vi "Read back eight strings from file.vi"(0 "File Path":path, 11 "error in (no error)":errorcluster) -> (2 "item 1":string, 3 "item 2":string, 4 "item 3":string, 6 "item 4":string, 8 "item 5":string, 10 "item 6":string, 13 "item 8":string, 14 "item 7":string, 15 "error out":errorcluster)   [LabVIEW 2013]
uses:
  <vilib>/Utility/file.llb/Read From Spreadsheet File (string).vi
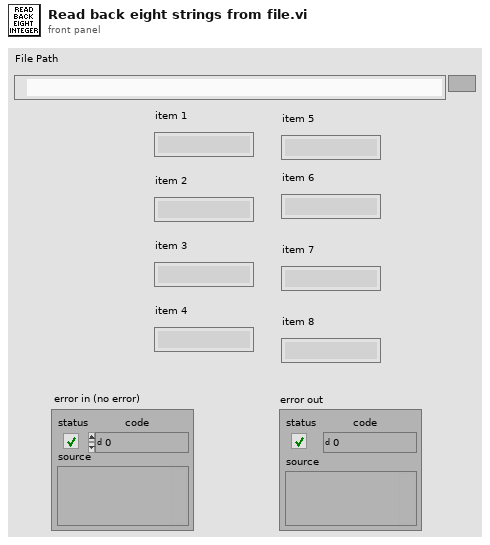
[diagram p1: front panel]
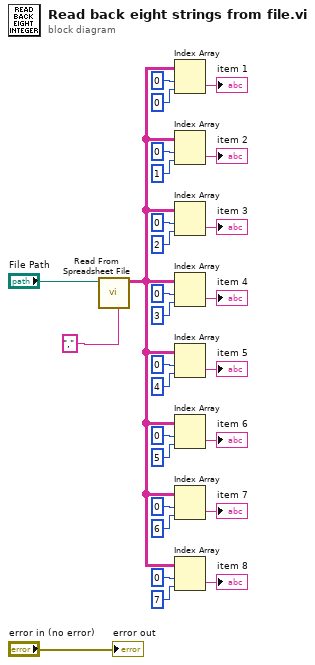
[diagram p0: block diagram]
diagram:
  n1 = call-poly <vilib>:"Read From Spreadsheet File.vi"("delimiter (\\t)"="," ("delimiter (\\t)"), "file path (dialog if empty)"="File Path") -> ("all rows"=w10:string[][])  [unwired: 5 in, 4 out]
  n2 = Index Array(array=w10, index (row)=0, index (col)=0 ("disabled index (col)")) -> (element=→"item 1":string)
  n3 = Index Array(array=w10, index (row)=0, index (col)=1 ("disabled index (col)")) -> (element=→"item 2":string)
  n4 = Index Array(array=w10, index (row)=0, index (col)=2 ("disabled index (col)")) -> (element=→"item 3":string)
  n5 = Index Array(array=w10, index (row)=0, index (col)=3 ("disabled index (col)")) -> (element=→"item 4":string)
  n6 = Index Array(array=w10, index (row)=0, index (col)=4 ("disabled index (col)")) -> (element=→"item 5":string)
  n7 = Index Array(array=w10, index (row)=0, index (col)=5 ("disabled index (col)")) -> (element=→"item 6":string)
  n8 = Index Array(array=w10, index (row)=0, index (col)=6 ("disabled index (col)")) -> (element=→"item 7":string)
  n9 = Index Array(array=w10, index (row)=0, index (col)=7 ("disabled index (col)")) -> (element=→"item 8":string)
  "error out" <- "error in (no error)"
